vi "Add Response_Wait sec.vi"(8 "Error In":errorcluster, 10 "Settings":T2 {"Linkages"."Linked Channel refnum" format="%.0x"; "Channel refnum" format="%.0x"}, 11 "Message Refnum In":T1=18446744073709551615 format="%.0x") -> (0 "Error Out":errorcluster, 2 "Response Refnum":T1=18446744073709551615 format="%.0x", 3 "Message Refnum Out":T1=18446744073709551615 format="%.0x")   [LabVIEW 2019, in "Scripting API.lvlib"]
uses:
  Scripting API.lvlib
  <vilib>/NI VeriStand/Custom Device API/Custom Device Item Ref.ctl
  Examples/Control 8.ctl
  <vilib>/NI VeriStand/Custom Device API/Custom Device API.lvlib
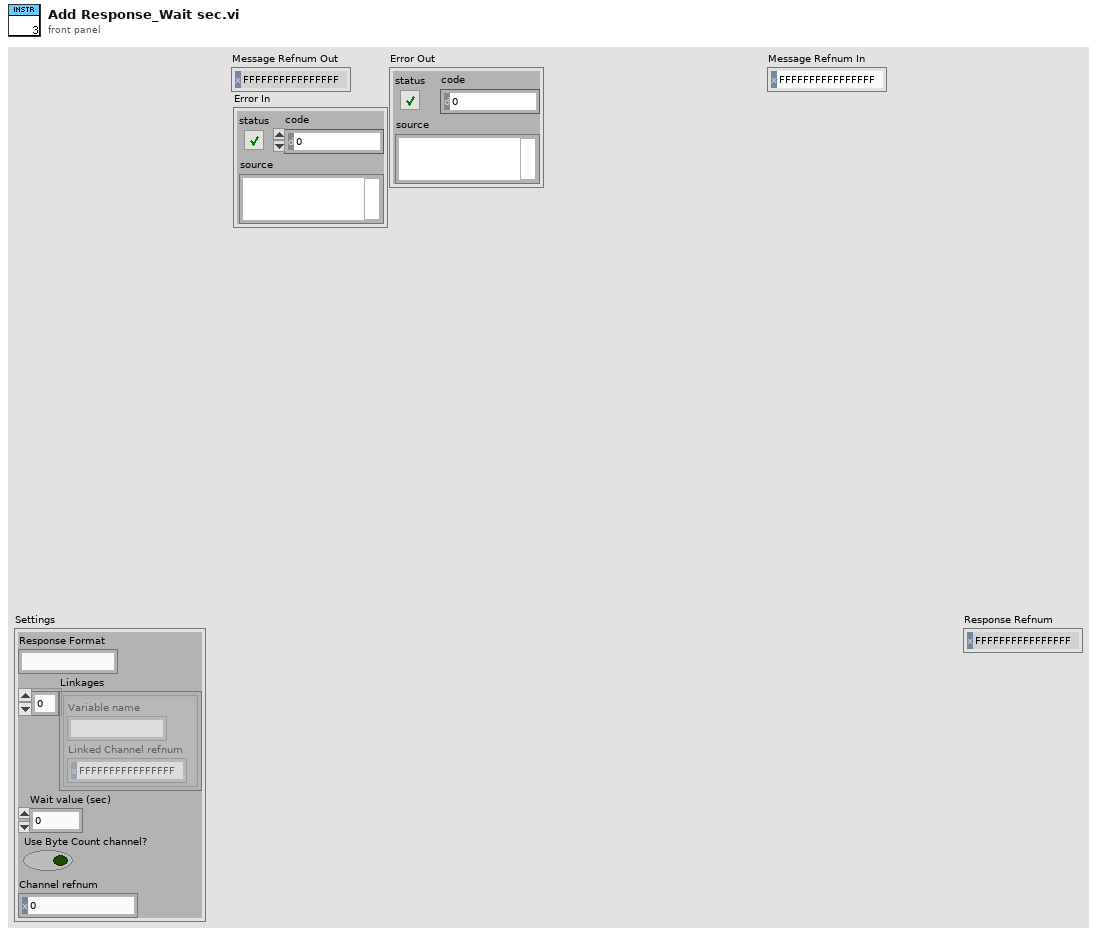
[diagram p1: front panel]
types:
  T1 = typedef "Custom Device API.lvlib/Custom Device Item Ref.ctl" = u64
  T2 = typedef "Control 8.ctl" = cluster{"Response Format":string, "Linkages":cluster{"Variable name":string, "Linked Channel refnum":T1}[], "Wait value (sec)":dbl, "Use Byte Count channel?":bool, "Channel refnum":T1}
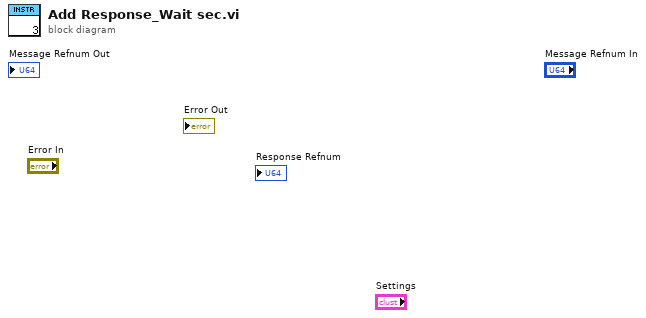
[diagram p0: block diagram]
diagram:
